vi "Firmware Wizard Config.vi"(8 "Error In":errorcluster) -> (0 "Error Out":errorcluster)   [LabVIEW 2014, in "LMH-LINX.lvlib"]
doc: "Allow user to configure settings stored in firmware wizard ini."
uses:
  <vilib>/MakerHub/LINX/LMH-LINX.lvlib
  <vilib>/Utility/config.llb/Read Key (Path).vi
  <vilib>/Utility/config.llb/Write Key (Path).vi
  <vilib>/Utility/config.llb/NI_LVConfig.lvlib
  <vilib>/MakerHub/Toolbox/LMH-Toolbox.lvlib
panel:
  in  "Generate Firmware Libs":bool
  in  "Arduino Path":path
  in  "Cancel Button":bool
  in  "Save Button":bool
  in  "LINX Firmware Base Path":path
  # "Default Location: <LabVIEW>\\vi.lib\\MakerHub\\LINX\\Firmware\\"
  # "Default Location: <Program Files (x86)>\\Arduino"
  # "If you have the Arduino IDE, fill in the Arduino Path and use the Generate button to Generate the LINX firmware in the Arduino\\libraries folder\nNOTE: This will erase existing LINX firmware in this folder"
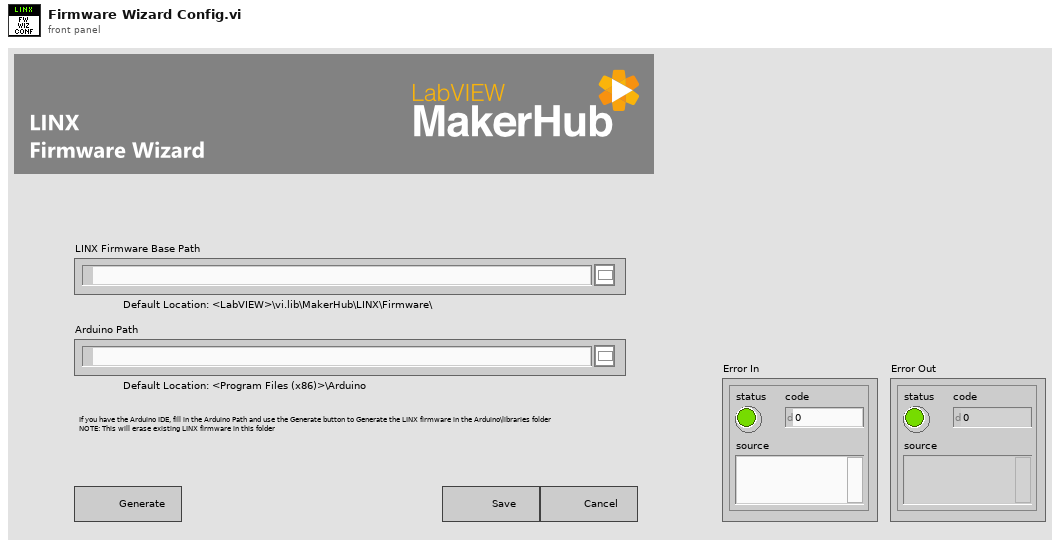
[diagram p1: front panel]
types:
  T1 = typedef "NI_LVConfig.lvlib/Config Data RefNum.ctl" = refnum<k1>
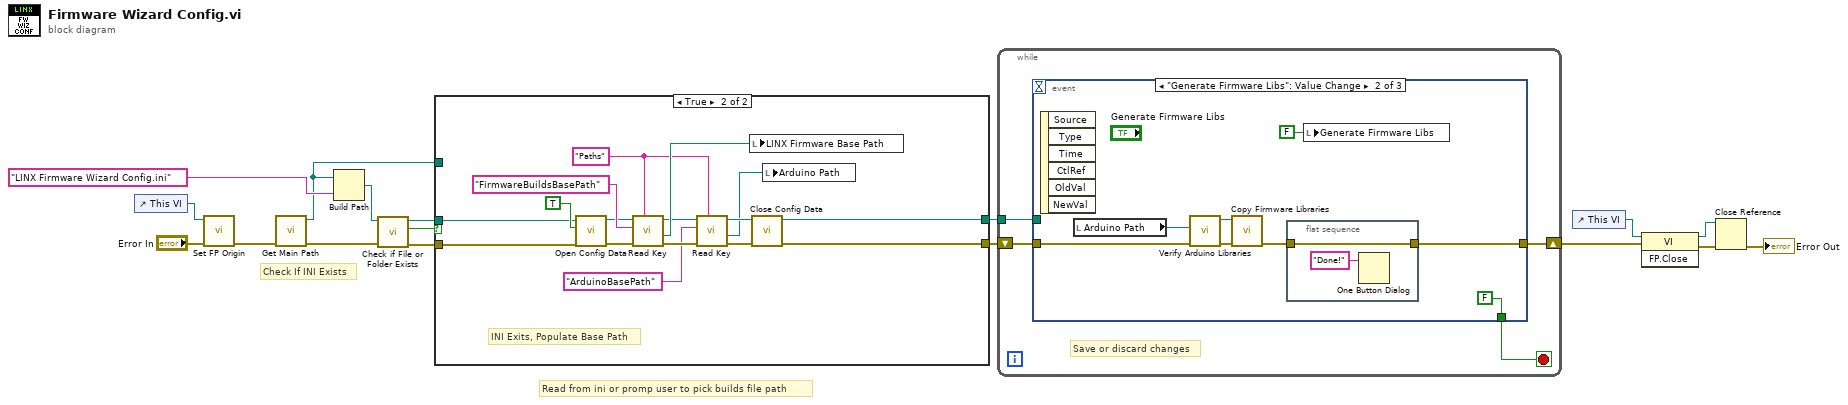
[diagram p0: block diagram]
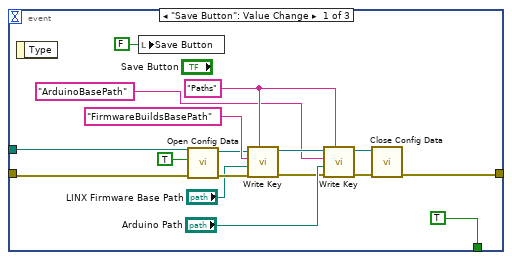
[diagram p2: hidden frame]
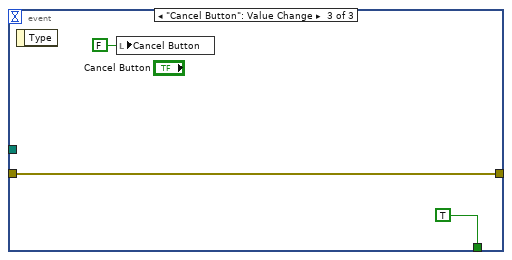
[diagram p3: hidden frame]
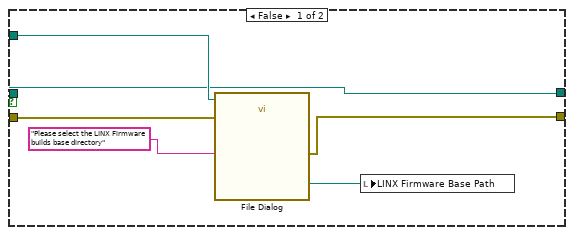
[diagram p4: hidden frame]
diagram:
  # "Read from ini or promp user to pick builds file path"
  # "Check If INI Exists"
  n1 = control-ref of="This VI"() -> (w8:refnum<vi>)
  n2 = call <vilib>:"Set FP Origin.vi"("Error In"="Error In", "VI Ref"=w8) -> ("Error Out"=w1:errorcluster)  [unwired: 9 in]
  n3 = call <vilib>:"Get Main Path.vi"("Error In"=w1) -> ("Error Out"=w16:errorcluster, "Main Dir"=w11:path)  [unwired: 8 in, 1 out]
  n4 = Build Path(base path=w11, name or relative path="LINX Firmware Wizard Config.ini") -> (appended path=w15:path)
  n5 = call <vilib>:"Check if File or Folder Exists.vi"("error in (no error)"=w16, "path"=w15) -> ("error out"=w12:errorcluster, "file or folder exists?"=w13:bool, "dup path"=w14:path)  [unwired: 7 in]
  n6 = case shown="True" w13 {
    tunnel: [w22 w35] -> w10
    tunnel: w14 -> [w20 w34]
    tunnel: w12 -> [w23 w33]
    tunnel: w11 -> [w21 _]
    tunnel: [w20 w32] -> w9
    frame False {
      n7 = call "File Dialog"("start path"=w21, "prompt"="Please select the LINX Firmware builds base directory", "error in"=w23) -> ("selected path"=w19:path, "error out"=w22:errorcluster)  [unwired: 9 in, 2 out]
      n8 = local write "LINX Firmware Base Path"(w19) -> ()
    }
    frame True {
      w28 = "Paths" ("section")
      # "INI Exits, Populate Base Path"
      n9 = call <vilib>:"Open Config Data.vi"("error in (no error)"=w33, "create file if necessary (T)"=TRUE, "configuration file path"=w34) -> ("error out"=w36:errorcluster, "refnum"=w37:T1)  [unwired: 6 in, 1 out]
      n10 = call-poly <vilib>:"Read Key.vi"("section"=w28, "error in (no error)"=w36, "key"="FirmwareBuildsBasePath", "refnum"=w37) -> ("error out"=w29:errorcluster, "value"=w31:path, "refnum out"=w30:T1)  [unwired: 4 in, 1 out]
      n11 = call-poly <vilib>:"Read Key.vi"("section"=w28, "error in (no error)"=w29, "key"="ArduinoBasePath", "refnum"=w30) -> ("error out"=w25:errorcluster, "value"=w24:path, "refnum out"=w26:T1)  [unwired: 4 in, 1 out]
      n12 = local write "LINX Firmware Base Path"(w31) -> ()
      n13 = call <vilib>:"Close Config Data.vi"("error in (no error)"=w25, "refnum"=w26) -> ("error out"=w35:errorcluster, "file path"=w32:path)  [unwired: 8 in]
      n14 = local write "Arduino Path"(w24) -> ()
    }
  }
  n15 = while {
    tunnel: w9 -> [w42]
    shift-right: [w41] -> w3
    shift-left: w10 -> [w43]
    stop <- w40 stop-if-true
    # "Save or discard changes"
    n16 = event shown="[1] \"Generate Firmware Libs\": Value Change" {
      selector: _ -> [_ _ _]
      dyn-events: _ -> [_ _ _]
      timeout: _ -> [_ _ _]
      tunnel: w43 -> [w58 w68 w72]
      tunnel: [w53 w62 w72] -> w41
      tunnel: w42 -> [w55 _ _]
      tunnel: [TRUE FALSE TRUE] -> w40
      event "Save Button": Value Change {
        w50 = "Paths" ("section")
        n17 = event-data() -> ()  [unwired: 1 in, 1 out]
        n18 = local write "Save Button"(FALSE ("Save Button")) -> ()
        n19 = call <vilib>:"Open Config Data.vi"("error in (no error)"=w58, "create file if necessary (T)"=TRUE, "configuration file path"=w55) -> ("error out"=w57:errorcluster, "refnum"=w54:T1)  [unwired: 6 in, 1 out]
        n20 = call-poly <vilib>:"Write Key.vi"("section"=w50, "error in (no error)"=w57, "value"="LINX Firmware Base Path", "key"="FirmwareBuildsBasePath", "refnum"=w54) -> ("error out"=w47:errorcluster, "refnum out"=w51:T1)  [unwired: 4 in, 1 out]
        n21 = call-poly <vilib>:"Write Key.vi"("section"=w50, "error in (no error)"=w47, "value"="Arduino Path", "key"="ArduinoBasePath", "refnum"=w51) -> ("error out"=w46:errorcluster, "refnum out"=w45:T1)  [unwired: 4 in, 1 out]
        n22 = call <vilib>:"Close Config Data.vi"("error in (no error)"=w46, "refnum"=w45) -> ("error out"=w53:errorcluster)  [unwired: 8 in, 1 out]
      }
      event "Generate Firmware Libs": Value Change {
        n23 = event-data() -> ()  [unwired: 1 in, 6 out]
        n24 = local read "Arduino Path"() -> (w67:path)
        n25 = call <vilib>:"Verify Arduino Libraries.vi"("Error In"=w68, "Arduino Base Path"=w67) -> ("Error Out"=w65:errorcluster, "Path to Arduino\\libraries"=w66:path)  [unwired: 7 in, 1 out]
        n26 = call <vilib>:"Copy Firmware Libraries.vi"("Error In"=w65, "Library Destination Dir"=w66) -> ("Error Out"=w61:errorcluster)  [unwired: 9 in]
        n27 = flat-sequence {
          tunnel: [w70] -> w62
          tunnel: w61 -> [w70]
          frame #0 {
            n28 = One Button Dialog(message="Done!") -> ()  [unwired: 1 in, 1 out]
          }
        }
        n29 = local write "Generate Firmware Libs"(FALSE ("Generate Firmware Libs")) -> ()
      }
      event "Cancel Button": Value Change {
        n30 = event-data() -> ()  [unwired: 1 in, 1 out]
        n31 = local write "Cancel Button"(FALSE ("Cancel Button")) -> ()
      }
    }
  }
  n32 = control-ref of="This VI"() -> (w4:refnum<vi>)
  n33 = invoke class="VI" method="FP.Close"(reference=w4, error in=w3) -> (reference out=w6:refnum<vi>, error out=w5:errorcluster)  [unwired: 1 in, 1 out]
  n34 = Close Reference(reference=w6, error in (no error)=w5) -> (error out=→"Error Out":errorcluster)
